vi "Write task.vi"(8 "error in (no error)":errorcluster, 10 "task":refnum<k21>, 11 "NI_DAQmx(Angular) in":refnum<class "NI_DAQmx(Angular).lvclass">) -> (0 "error out":errorcluster, 3 "NI_DAQmx(Angular) out":refnum<class "NI_DAQmx(Angular).lvclass">)   [LabVIEW 2025, in "NI_DAQmx(Angular).lvclass"]
uses:
  NI_DAQmx(Angular).lvclass
  NI_DAQmx(Angular).lvclass/NI_DAQmx(Angular).ctl
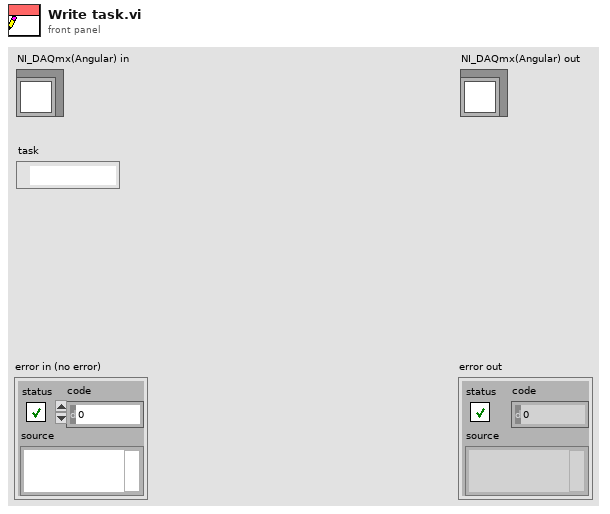
[diagram p1: front panel]
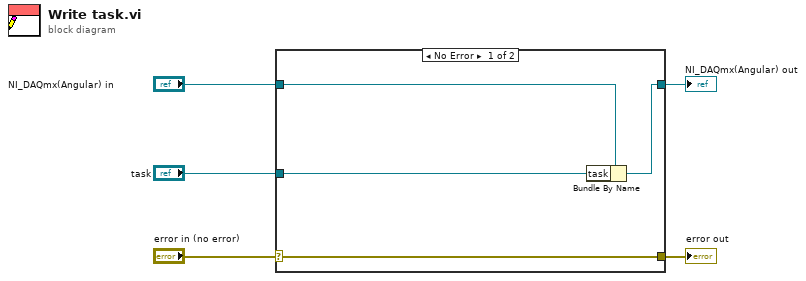
[diagram p0: block diagram]
diagram:
  n1 = case shown="No Error" "error in (no error)" {
    selector: "error in (no error)" -> [w9 w10]
    tunnel: [w9 w10] -> w4
    tunnel: [w7 w11] -> w2
    tunnel: "NI_DAQmx(Angular) in" -> [w8 w11]
    tunnel: "task" -> [w6 _]
    frame No Error {
      n2 = Bundle By Name(cluster=w8, "task"=w6) -> (w7:refnum<class "NI_DAQmx(Angular).lvclass">)
    }
    frame Error {
    }
  }
  "error out" <- w4
  "NI_DAQmx(Angular) out" <- w2
